vi "Model In Caller.vi"(8 "error in (no error)":errorcluster caption="Error In") -> (0 "error out":errorcluster caption="Error Out")   [LabVIEW 2020]
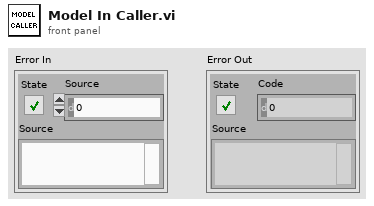
[diagram p1: front panel]
types:
  T1 = enum32{"Invalid", "Default", "Floating", "Floating/Auto-Hide", "Modal"}
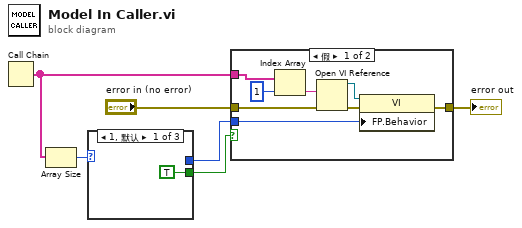
[diagram p0: block diagram]
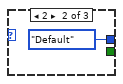
[diagram p3: hidden frame]
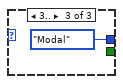
[diagram p4: hidden frame]
diagram:
  n1 = Call Chain() -> (call chain=w4:string[])
  n2 = Array Size(array=w4) -> (size(s)=w6:i32)
  n3 = case shown="1, 默认" w6 {
    tunnel: [TRUE _ _] -> w5
    tunnel: [_ T1."Default" ("前面板窗口:动作") T1."Modal" ("前面板窗口:动作")] -> w3
    frame 1, Default {
    }
    frame 2 {
    }
    frame 3.. {
    }
  }
  n4 = case shown="假" w5 {
    tunnel: w4 -> [w16 _]
    tunnel: w3 -> [w13 _]
    tunnel: "error in (no error)" -> [w12 w18]
    tunnel: [w10 w18] -> w1
    frame False {
      n5 = Index Array(array=w16, index=1 ("索引")) -> (element=w15:string)
      n6 = Open VI Reference(vi path=w15, error in (no error)=w12) -> (vi reference=w14:refnum<vi>, error out=w11:errorcluster)  [unwired: 4 in]
      n7 = property class="VI"(reference=w14, error in=w11, "FP.Behavior"=w13) -> (error out=w10:errorcluster)  [unwired: 1 out]
    }
    frame True {
    }
  }
  "error out" <- w1
